vi "Pre Launch Init.vi"(11 "KeysightN9020B in":refnum<class "KeysightN9020B.lvclass">) -> (0 "error out":errorcluster, 3 "KeysightN9020B out":refnum<class "KeysightN9020B.lvclass">)   [LabVIEW 2023, in "KeysightN9020B.lvlib" / "KeysightN9020B.lvclass"]
doc: "(<B>Filename</B>: Actor Framework.lvlib:Actor.lvclass:Pre Launch Init.vi)\n\nDefines behavior that occurs after the Launch Nested Actor method is invoked but before the actor's Actor Core method begins running.\n\nBy default, this method does nothing. A descendant class may override it to define behavior."
uses:
  KeysightN9020B.lvclass
  KeysightN9020B.lvclass/KeysightN9020B.ctl
  <vilib>/ActorFramework/Actor/Actor.lvclass
panel:
  in  "Array":dbl[][](array[numeric])
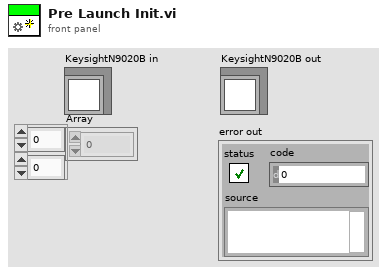
[diagram p1: front panel]
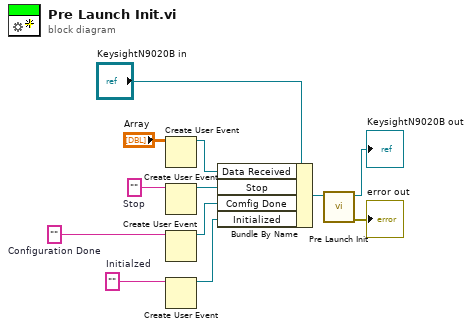
[diagram p0: block diagram]
diagram:
  w8 = ""  # Configuration Done
  w9 = ""  # Initialzed
  w10 = ""  # Stop
  n1 = Create User Event(user event datatype="Array") -> (user event=w1:refnum<user-event>)  [unwired: 1 in, 1 out]
  n2 = Create User Event(user event datatype=w10) -> (user event=w5:refnum<user-event>)  [unwired: 1 in, 1 out]
  n3 = Create User Event(user event datatype=w8) -> (user event=w3:refnum<user-event>)  [unwired: 1 in, 1 out]
  n4 = Create User Event(user event datatype=w9) -> (user event=w4:refnum<user-event>)  [unwired: 1 in, 1 out]
  n5 = Bundle By Name(cluster="KeysightN9020B in", "Data Received"=w1, "Stop"=w5, "Comfig Done"=w3, "Initialized"=w4) -> (w6:refnum<class "KeysightN9020B.lvclass">)
  n6 = call-parent "Pre Launch Init.vi"("Actor in"=w6) -> ("error out"=→"error out":errorcluster, "Actor out"=→"KeysightN9020B out":refnum<class "KeysightN9020B.lvclass">)  [unwired: 9 in]
